vi "Search_dust_names.vi"(8 "error in (no error)":errorcluster, 11 "Dust array in":T1[](array[typedef])) -> (0 "error out":errorcluster, 2 "Cancelled?":bool, 3 "Dust array out":T1[](array[typedef]))   [LabVIEW 2013]
uses:
  Controls/Dust_list.ctl
  <vilib>/Utility/miscctls.llb/LVPointTypeDef.ctl
panel:
  in  "Get All":bool
  in  "Cancel":bool
  in  "Select":bool
  in  "Search":bool
  in  "Search Name":string
  out "Dust Name Array":string[](array[string])
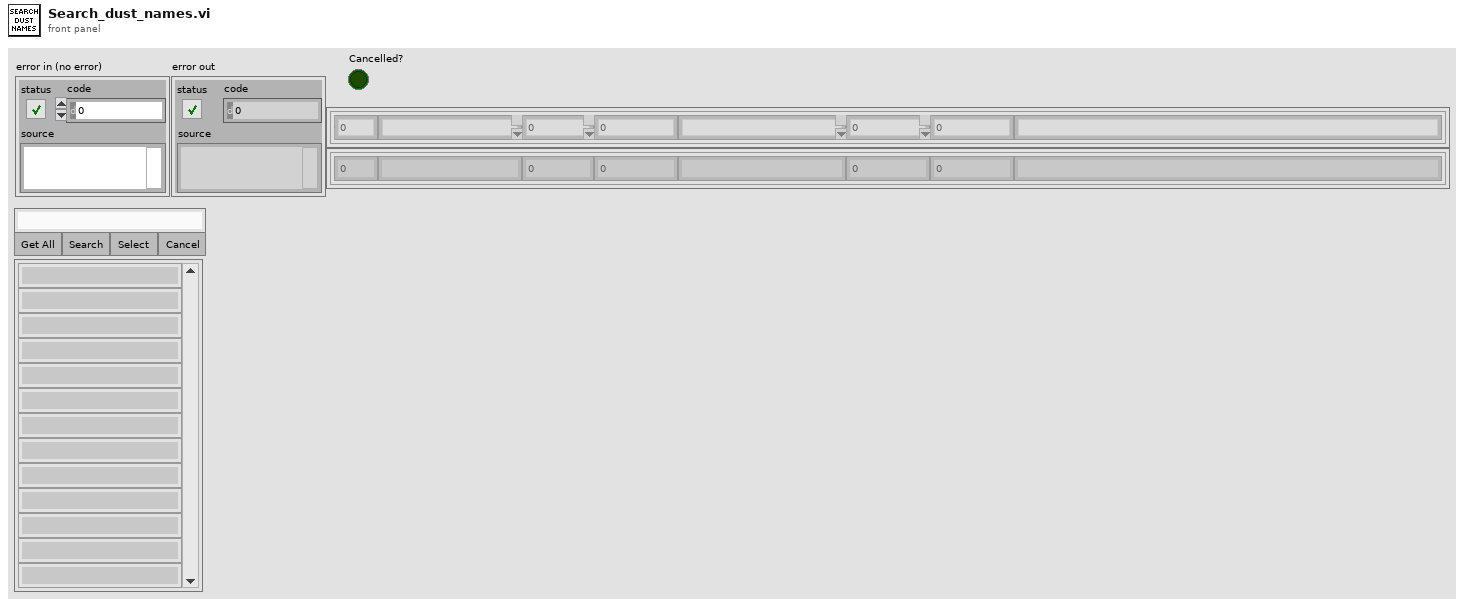
[diagram p1: front panel]
types:
  T1 = typedef "dust_list.ctl" = cluster{"id_dust_type":i32, "dust_name":string, "dust_density":dbl, "source_weight":dbl, "size":string, "bottle_weight":dbl, "dust_mass":dbl, "comments":string}
  T2 = enum16{"dust_name", "dust_density", "source_weight", "bottle_weight", "dust_weight"}
  T3 = typedef "LVPointTypeDef.ctl" = cluster{"Horizontal":i16, "Vertical":i16}
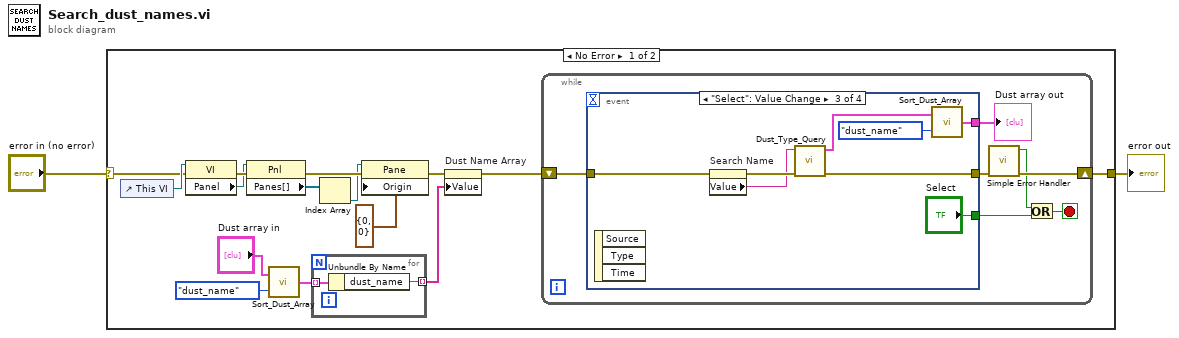
[diagram p0: block diagram]
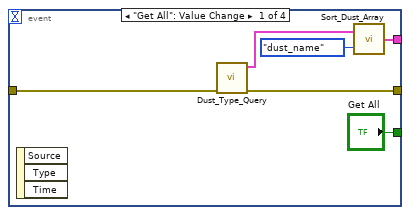
[diagram p2: hidden frame]
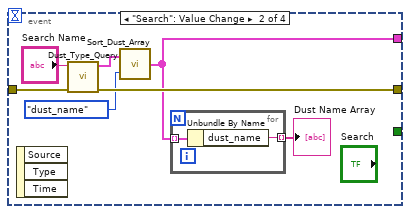
[diagram p3: hidden frame]
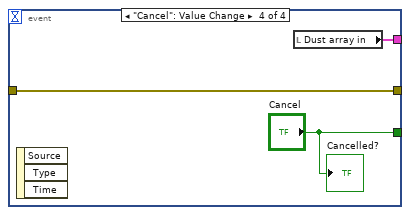
[diagram p4: hidden frame]
diagram:
  n1 = case shown="No Error" "error in (no error)" {
    selector: "error in (no error)" -> [w8 w53]
    tunnel: [w7 w53] -> w1
    frame No Error {
      n2 = control-ref of="This VI"() -> (w15:refnum<vi>)
      n3 = property class="VI"(reference=w15, error in=w8) -> (error out=w14:errorcluster, "Panel"=w13:refnum<vi>)  [unwired: 1 out]
      n4 = property class="Pnl"(reference=w13, error in=w14) -> (error out=w12:errorcluster, "Panes[]"=w11:refnum<vi>[])  [unwired: 1 out]
      n5 = call "Sort_Dust_Array.vi"("Order by..."=T2."dust_name", "Array In"="Dust array in") -> ("Array out"=w3:T1[])
      n6 = for {
        tunnel: w3 -> [w52] mode=indexing
        tunnel: [w51] -> w6 mode=indexing
        n7 = Unbundle By Name(w52) -> ("dust_name"=w51:string)
      }
      n8 = Index Array(array=w11) -> (element=w10:refnum<vi>)  [unwired: 1 in]
      n9 = property class="Pane"(reference=w10, error in=w12, "Origin"=T3 {"Horizontal"=0, "Vertical"=0}) -> (error out=w16:errorcluster)  [unwired: 1 out]
      n10 = property on="Dust Name Array" class="Arr (strict)"(error in=w16, "Value"=w6) -> (error out=w17:errorcluster)  [unwired: 1 in, 1 out]
      n11 = while {
        shift-right: [w21] -> w7
        shift-left: w17 -> [w23]
        stop <- w20 stop-if-true
        n12 = event shown="[2] \"Select\": Value Change" {
          selector: _ -> [_ _ _ _]
          dyn-events: _ -> [_ _ _ _]
          timeout: _ -> [_ _ _ _]
          tunnel: [w29 w37 w46 w50] -> w24
          tunnel: w23 -> [w30 w35 w43 w50]
          tunnel: ["Get All" _ "Select" "Cancel"] -> w22
          tunnel: [w26 w31 w41 w48] -> w18
          event "Get All": Value Change {
            n13 = event-data() -> ()  [unwired: 1 in, 3 out]
            n14 = call "Dust_Type_Query.vi"("error in (no error)"=w30) -> ("error out"=w29:errorcluster, "Dust Type Array"=w25:T1[])  [unwired: 9 in]
            n15 = call "Sort_Dust_Array.vi"("Order by..."=T2."dust_name", "Array In"=w25) -> ("Array out"=w26:T1[])
          }
          event "Search": Value Change {
            n16 = event-data() -> ()  [unwired: 1 in, 3 out]
            n17 = call "Dust_Type_Query.vi"("error in (no error)"=w35, "Dust Name"="Search Name") -> ("error out"=w37:errorcluster, "Dust Type Array"=w32:T1[])  [unwired: 8 in]
            n18 = call "Sort_Dust_Array.vi"("Order by..."=T2."dust_name", "Array In"=w32) -> ("Array out"=w31:T1[])
            n19 = for {
              tunnel: [w39] -> w34 mode=indexing
              tunnel: w31 -> [w38] mode=indexing
              n20 = Unbundle By Name(w38) -> ("dust_name"=w39:string)
            }
            "Dust Name Array" <- w34
          }
          event "Select": Value Change {
            n21 = event-data() -> ()  [unwired: 1 in, 3 out]
            n22 = property on="Search Name" class="Str"(error in=w43) -> (error out=w45:errorcluster, "Value"=w44:string)  [unwired: 1 in, 1 out]
            n23 = call "Dust_Type_Query.vi"("error in (no error)"=w45, "Dust Name"=w44) -> ("error out"=w46:errorcluster, "Dust Type Array"=w40:T1[])  [unwired: 8 in]
            n24 = call "Sort_Dust_Array.vi"("Order by..."=T2."dust_name", "Array In"=w40) -> ("Array out"=w41:T1[])
          }
          event "Cancel": Value Change {
            n25 = event-data() -> ()  [unwired: 1 in, 3 out]
            n26 = local read "Dust array in"() -> (w48:T1[])
            "Cancelled?" <- "Cancel"
          }
        }
        "Dust array out" <- w18
        n27 = call <vilib>:"Simple Error Handler.vi"("error in (no error)"=w24) -> ("error?"=w19:bool, "error out"=w21:errorcluster)  [unwired: 4 in, 3 out]
        n28 = Or(x=w19, y=w22) -> (x .or. y?=w20:bool)
      }
    }
    frame Error {
    }
  }
  "error out" <- w1
